vi "Eval Test.vi"(8 "error in (no error)":errorcluster, 11 "Plugin_Controller in":refnum<class "Plugin_Controller.lvclass">) -> (0 "error out":errorcluster, 1 "Passed?":bool[](array[boolean]), 2 "Result String":string[][](array[string]), 3 "Plugin_Controller out":refnum<class "Plugin_Controller.lvclass">)   [LabVIEW 2020, in "Plugin.lvlib" / "Plugin_UI.lvclass"]
doc: "Parse the result and format the Result table data."
uses:
  Plugin_UI.lvclass
  Controller_Class/Plugin_Controller.lvclass
  C:/SVN_LabSys/labsys_lvcode/LabSys_SourceCode/builds/Libraries/LabSys Framework.lvlibp/Data Node/Data Node/Data Node.lvclass
  C:/SVN_LabSys/labsys_lvcode/LabSys_SourceCode/builds/Libraries/LabSys Framework.lvlibp/Configurable Data Node/Configurable Data Node/Configurable Data Node.lvclass
  builds/Libraries/LabSys Framework.lvlibp/Configuration Storage/Test Configuration/Test Configuration.lvclass
  builds/Libraries/LabSys Framework.lvlibp/Data Distributor/Value/Value Status.ctl
  builds/Libraries/LabSys Framework.lvlibp/Data Distributor/Data Distributor/Data Distributor.lvclass
  builds/Libraries/LabSys Framework.lvlibp/Data Node/Data Node/Read Data Distributor.vi
  builds/Libraries/LabSys Framework.lvlibp/Configurable Data Node/Configurable Data Node/Read Module Configuration.vi
  builds/Libraries/LabSys Framework.lvlibp/Configuration Storage/Module Configuration/Read Test Configuration.vi
  builds/Libraries/LabSys Framework.lvlibp/Data Distributor/Value/Read Time Stamp.vi
  builds/Libraries/LabSys Framework.lvlibp/Data Distributor/Value/Read Status.vi
  builds/Libraries/LabSys Framework.lvlibp/Configuration Storage/Module Configuration/Module Configuration.lvclass
  builds/Libraries/LabSys Framework.lvlibp/Data Distributor/Value/Value.lvclass
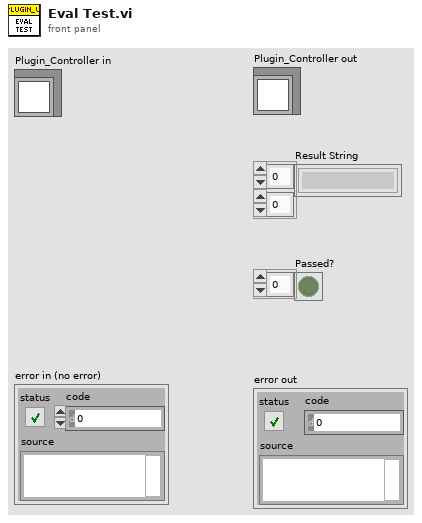
[diagram p1: front panel]
types:
  T1 = typedef "LabSys Framework.lvlibp/Data Distributor.lvlib/Value.lvclass/Value Status.ctl" = enum8{"FAIL", "OK", "UNDEFINED"}
  T2 = typedef "LabSys Framework.lvlibp/Configuration Storage.lvlib/Test Configuration.lvclass/Channel Information.ctl" = cluster{"Channel Direction":T3, "Alias":string, "Refresh (ms)":dbl, "Scaling Information":T4, "Value Type":T6, "Subchannels":T7[], "Auxiliary Data":variant, "Group":i32}
  T3 = typedef "LabSys Framework.lvlibp/Configuration Storage.lvlib/Test Configuration.lvclass/Channel Directions.ctl" = enum8{"Module Input", "Module Output"}
  T4 = typedef "LabSys Framework.lvlibp/Configuration Storage.lvlib/Test Configuration.lvclass/Scaling Information.ctl" = cluster{"Active":bool, "Scaling Type":T5, "Output Minimum":dbl, "Output Maximum":dbl, "Raw Minimum":dbl, "Raw Maximum":dbl, "Output Unit":string, "Function":string, "Lookup Table":string}
  T5 = typedef "LabSys Framework.lvlibp/Configuration Storage.lvlib/Test Configuration.lvclass/Scaling Types.ctl" = enum8{"Linear", "Function", "Lookup Table"}
  T6 = typedef "Framework Base Library.lvlibp/Value Types.ctl" = enum8{"Unknown", "double", "double array", "Waveform", "DigWaveform", "Boolean", "Decimal", "String", "Db2Message", "Byte Array", "Unsigned Decimal"}
  T7 = typedef "LabSys Framework.lvlibp/Configuration Storage.lvlib/Test Configuration.lvclass/Subchannel Information.ctl" = cluster{"Alias":string, "Start Bit":u32, "Bit Length":u32, "Value Type":T6, "Auxiliary Data":variant}
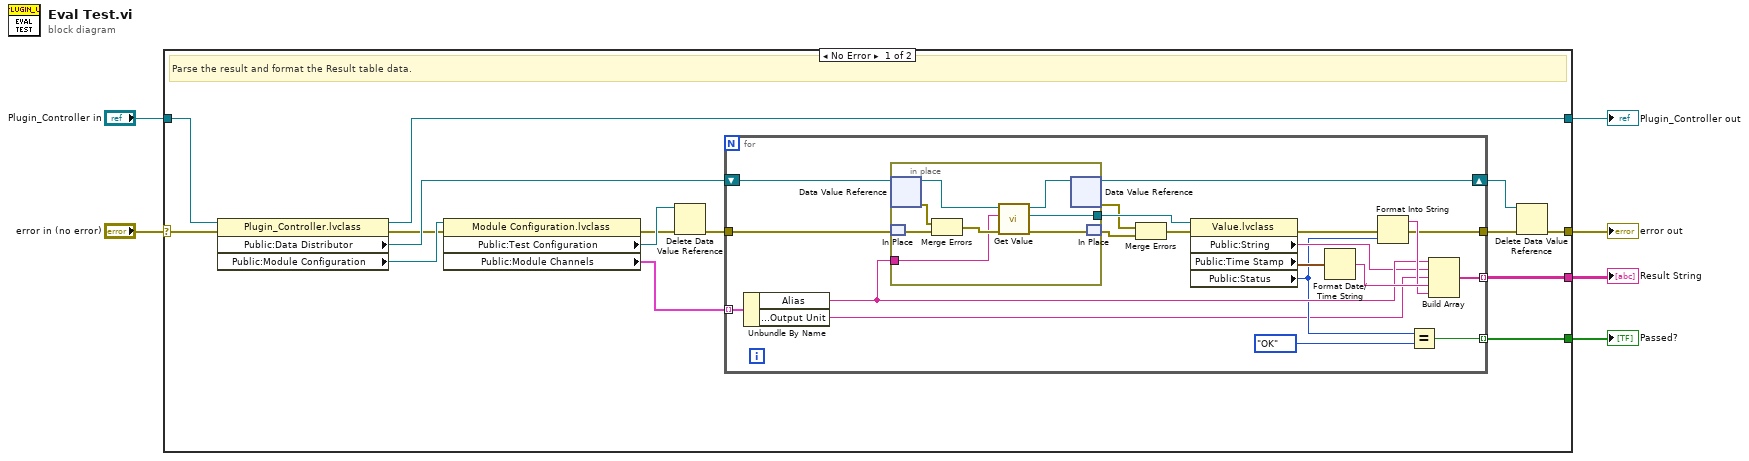
[diagram p0: block diagram]
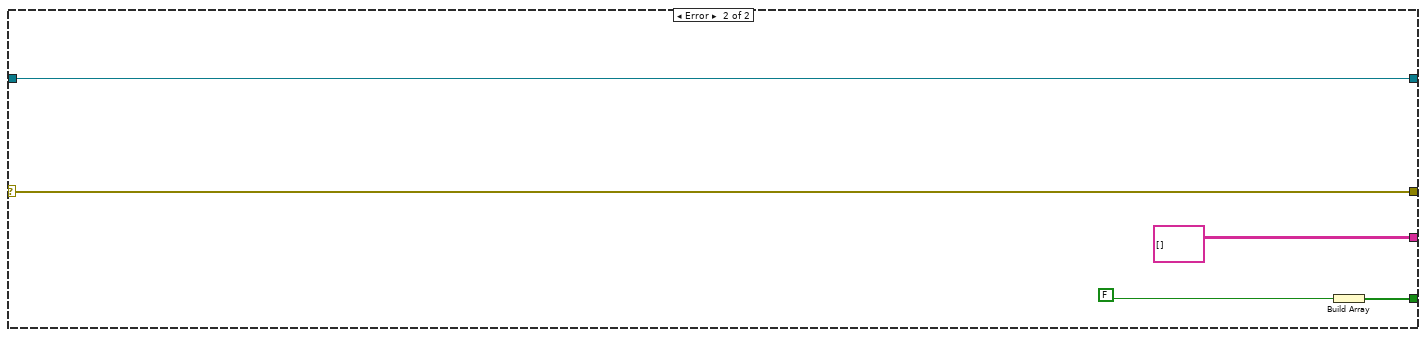
[diagram p2: hidden frame]
diagram:
  n1 = case shown="No Error" "error in (no error)" {
    selector: "error in (no error)" -> [w21 w53]
    tunnel: "Plugin_Controller in" -> [w17 w54]
    tunnel: [w16 w54] -> w4
    tunnel: [w7 w53] -> w3
    tunnel: [w15 string[][] []] -> w2
    tunnel: [w14 w50] -> w1
    frame No Error {
      # "Parse the result and format the Result table data."
      n2 = property class="Plugin_Controller.lvclass"(reference=w17, error in=w21) -> (reference out=w16:refnum<class "Plugin_Controller.lvclass">, error out=w13:errorcluster, "Public:Data Distributor"=w19:refnum<data-value>, "Public:Module Configuration"=w18:refnum<class "Module Configuration.lvclass">)
      n3 = property class="Module Configuration.lvclass"(reference=w18, error in=w13) -> (error out=w11:errorcluster, "Public:Test Configuration"=w12:refnum<data-value>, "Public:Module Channels"=w20:T2[])  [unwired: 1 out]
      n4 = Delete Data Value Reference(data value reference=w12, error in=w11) -> (error out=w10:errorcluster)  [unwired: 1 out]
      n5 = for {
        tunnel: [w35] -> w14 mode=indexing
        tunnel: [w34] -> w15 mode=indexing
        tunnel: [w24] -> w8
        tunnel: w20 -> [w30] mode=indexing
        tunnel: w10 -> [w28]
        shift-right: [w27] -> w9
        shift-left: w19 -> [w41]
        n6 = Unbundle By Name(w30) -> ("Alias"=w29:string, "Scaling Information.Output Unit"=w22:string)
        n7 = in-place {
          in-place-border: [w47] -> w40
          in-place-border: w29 -> [w42]
          n8 = in-place-dvr #1(w41) -> (w49:refnum<class "Data Distributor.lvclass">, w45:errorcluster)
          n9 = in-place-match #2(w28) -> (w44:errorcluster)
          n10 = Merge Errors(w45, w44) -> (w43:errorcluster)
          n11 = call-dynamic "Get Value.vi"("error in (no error)"=w43, "Variable Name"=w42, "Data Distributor in"=w49) -> ("error out"=w46:errorcluster, "Value"=w47:refnum<class "Value.lvclass">, "Data Distributor out"=w48:refnum<class "Data Distributor.lvclass">)  [unwired: 6 in]
          n12 = in-place-dvr #1(w48) -> (w27:refnum<data-value>, w32:errorcluster)
          n13 = in-place-match #2(w46) -> (w33:errorcluster)
        }
        n14 = Merge Errors(w32, w33) -> (w31:errorcluster)
        n15 = property class="Value.lvclass"(reference=w40, error in=w31) -> (error out=w25:errorcluster, "Public:String"=w26:string, "Public:Time Stamp"=w36:timestamp, "Public:Status"=w23:T1)  [unwired: 1 out]
        n16 = Format Date/Time String(seconds (now)=w36) -> (date/time string=w39:string)  [unwired: 2 in]
        n17 = Format Into String(error in=w25, w23) -> (resulting string=w38:string, error out=w24:errorcluster)  [unwired: 2 in]
        n18 = Equal?(x=w23, y=Value_Status."OK") -> (x = y?=w35:bool)
        n19 = Build Array(w29, w26, w22, w39, w38) -> (w34:string[])
      }
      n20 = Delete Data Value Reference(data value reference=w9, error in=w8) -> (error out=w7:errorcluster)  [unwired: 1 out]
    }
    frame Error {
      n21 = Build Array(FALSE) -> (w50:bool[])
    }
  }
  "Plugin_Controller out" <- w4
  "error out" <- w3
  "Result String" <- w2
  "Passed?" <- w1
